vi "resize table.vi"(8 "error in (no error)":errorcluster, 9 "Column Weights":i32[](array[numeric]), 10 "table":refnum<vi>, 11 "Pane in":refnum<vi>) -> (0 "error out":errorcluster)   [LabVIEW 2016, in "FPGA Resource Manager.lvlib"]
uses:
  FPGA Resource Manager.lvlib
  <vilib>/Utility/miscctls.llb/LVRowAndColumnTypeDef.ctl
  Shared/global constants.vi
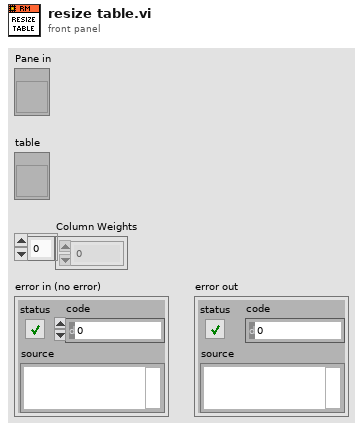
[diagram p1: front panel]
types:
  T1 = typedef "LVRowAndColumnTypeDef.ctl" = cluster{"Row":i32, "Column":i32}
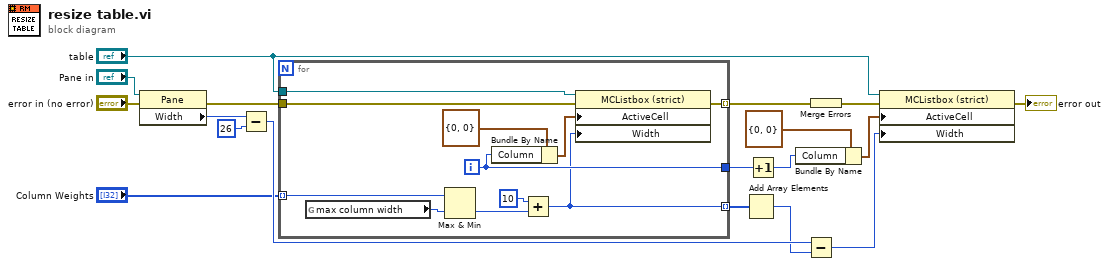
[diagram p0: block diagram]
diagram:
  n1 = property class="Pane"(reference="Pane in", error in="error in (no error)") -> (error out=w4:errorcluster, "Width"=w10:u32)  [unwired: 1 out]
  n2 = Subtract(x=w10, y=u32 26 ("x")) -> (x-y=w17:u32)
  n3 = for {
    tunnel: "Column Weights" -> [w23] mode=indexing
    tunnel: "table" -> [w29]
    tunnel: [w20] -> w8 mode=indexing
    tunnel: [w26] -> w11
    tunnel: w4 -> [w25]
    tunnel: [w24] -> w3 mode=indexing
    i -> [w26]
    n4 = global read "global constants.vi" "max column width"() -> (w22:i32)
    n5 = Max & Min(x=w23, y=w22) -> (min(x,y)=w21:i32)  [unwired: 1 out]
    n6 = Bundle By Name(cluster=T1 {"Row"=0, "Column"=0} ("Active Cell:Active Cell"), "Column"=w26) -> (w27:T1)
    n7 = Add(x=10, y=w21) -> (x+y=w20:i32)
    n8 = property class="MCListbox (strict)"(reference=w29, error in=w25, "ActiveCell"=w27, "Width"=w20) -> (error out=w24:errorcluster)  [unwired: 1 out]
  }
  n9 = Add Array Elements(numeric array=w8) -> (sum=w9:i32)
  n10 = Increment(x=w11) -> (x+1=w12:i32)
  n11 = Bundle By Name(cluster=T1 {"Row"=0, "Column"=0} ("Active Cell:Active Cell"), "Column"=w12) -> (w13:T1)
  n12 = Subtract(x=w17, y=w9) -> (x-y=w15:u32)
  n13 = Merge Errors(w3) -> (w2:errorcluster)
  n14 = property class="MCListbox (strict)"(reference="table", error in=w2, "ActiveCell"=w13, "Width"=w15) -> (error out=→"error out":errorcluster)  [unwired: 1 out]
